vi "stage1.vi"() -> (0 "pass":bool=TRUE, 1 "Boolean 5":bool, 2 "Boolean 8":bool, 3 "Boolean 7":bool)   [LabVIEW 2014]
uses:
  <vilib>/Utility/miscctls.llb/LVPositionTypeDef.ctl
panel:
  out "star 3":bool
  out "star 2":bool
  out "star 1":bool
  out "result":bool
  in  "hh":dbl format="%0#2_6g"
  in  ":":dbl format="%0#2_6g"
  in  "ss":dbl format="%0#2_6g"
  in  "Position 2":T1={"Left"=876, "Top"=156}
  in  "Boolean 6":bool
  out "Boolean 3":bool
  out "Boolean":bool
  out "Boolean 2":bool
  in  "OK Button 43":bool
  in  "Position":T1
  in  "character":bool
  out "Map Array 2":bool[][](array[boolean])
  in  "Map Array":dbl[][](array[numeric])=array130x130[16900 elements]
  in  "OK Button 42":bool
  in  "OK Button 41":bool
  in  "OK Button 40":bool
  in  "OK Button 39":bool
  in  "OK Button 38":bool
  in  "OK Button 37":bool
  in  "OK Button 36":bool
  in  "OK Button 35":bool
  in  "OK Button 34":bool
  in  "OK Button 33":bool
  in  "OK Button 32":bool
  in  "OK Button 31":bool
  in  "OK Button 30":bool
  in  "OK Button 29":bool
  in  "OK Button 28":bool
  in  "OK Button 27":bool
  in  "OK Button 26":bool
  in  "OK Button 25":bool
  in  "OK Button 24":bool
  in  "OK Button 23":bool
  in  "OK Button 22":bool
  in  "OK Button 21":bool
  in  "stop 6":bool
  in  "OK Button 20":bool
  in  "OK Button 19":bool
  in  "OK Button 18":bool
  in  "OK Button 17":bool
  in  "OK Button 16":bool
  in  "OK Button 15":bool
  in  "OK Button 14":bool
  in  "OK Button 13":bool
  in  "OK Button 12":bool
  in  "OK Button 11":bool
  in  "stop 5":bool
  in  "stop 4":bool
  in  "OK Button 10":bool
  in  "OK Button 9":bool
  in  "OK Button 8":bool
  in  "OK Button 7":bool
  in  "OK Button 6":bool
  in  "OK Button 5":bool
  in  "stop 3":bool
  in  "stop 2":bool
  in  "stop":bool
  in  "OK Button 4":bool
  in  "OK Button 3":bool
  in  "OK Button 2":bool
  in  "OK Button":bool
  out "Boolean 4":bool
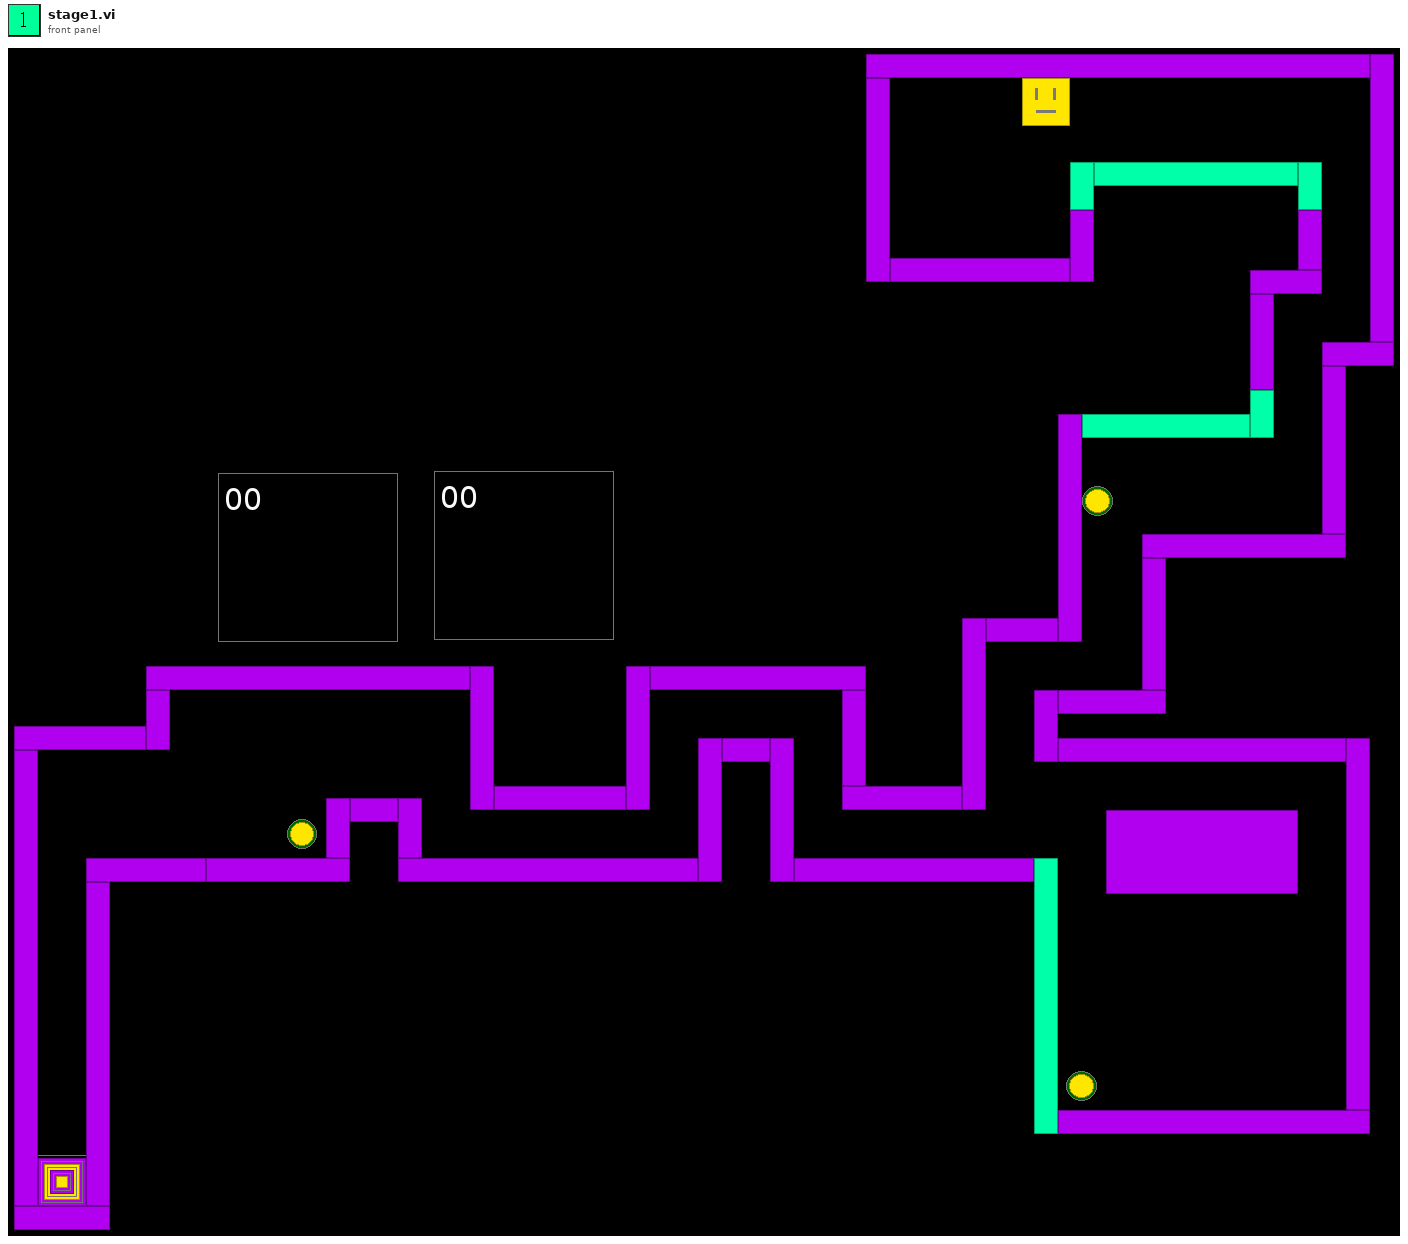
[diagram p1: front panel]
types:
  T1 = typedef "LVPositionTypeDef.ctl" = cluster{"Left":i32, "Top":i32}
  T2 = typedef "eventvkey.ctl" = enum16{"ASCII", "Enter", "Return", "Shift", "Ctrl", "Alt", "Cmd", "Opt", "Caps", "NumLock", "Clear", "Break", "Up", "Down", "Left", "Right", "Insert", "Delete", "Home", "End", "PageUp", "PageDown", "Escape", "Help", "Pause", "ScrollLock", "F1", "F2", "F3", "F4", "F5", "F6", "F7", "F8", "F9", "F10", "F11", "F12", "F13", "F14", "F15", "F16", "F17", "F18", "F19", "F20", "F21", "F22", "F23", "F24", "Play", "VolumeUp", "VolumeDown", "Mute", "Two Byte Char"}
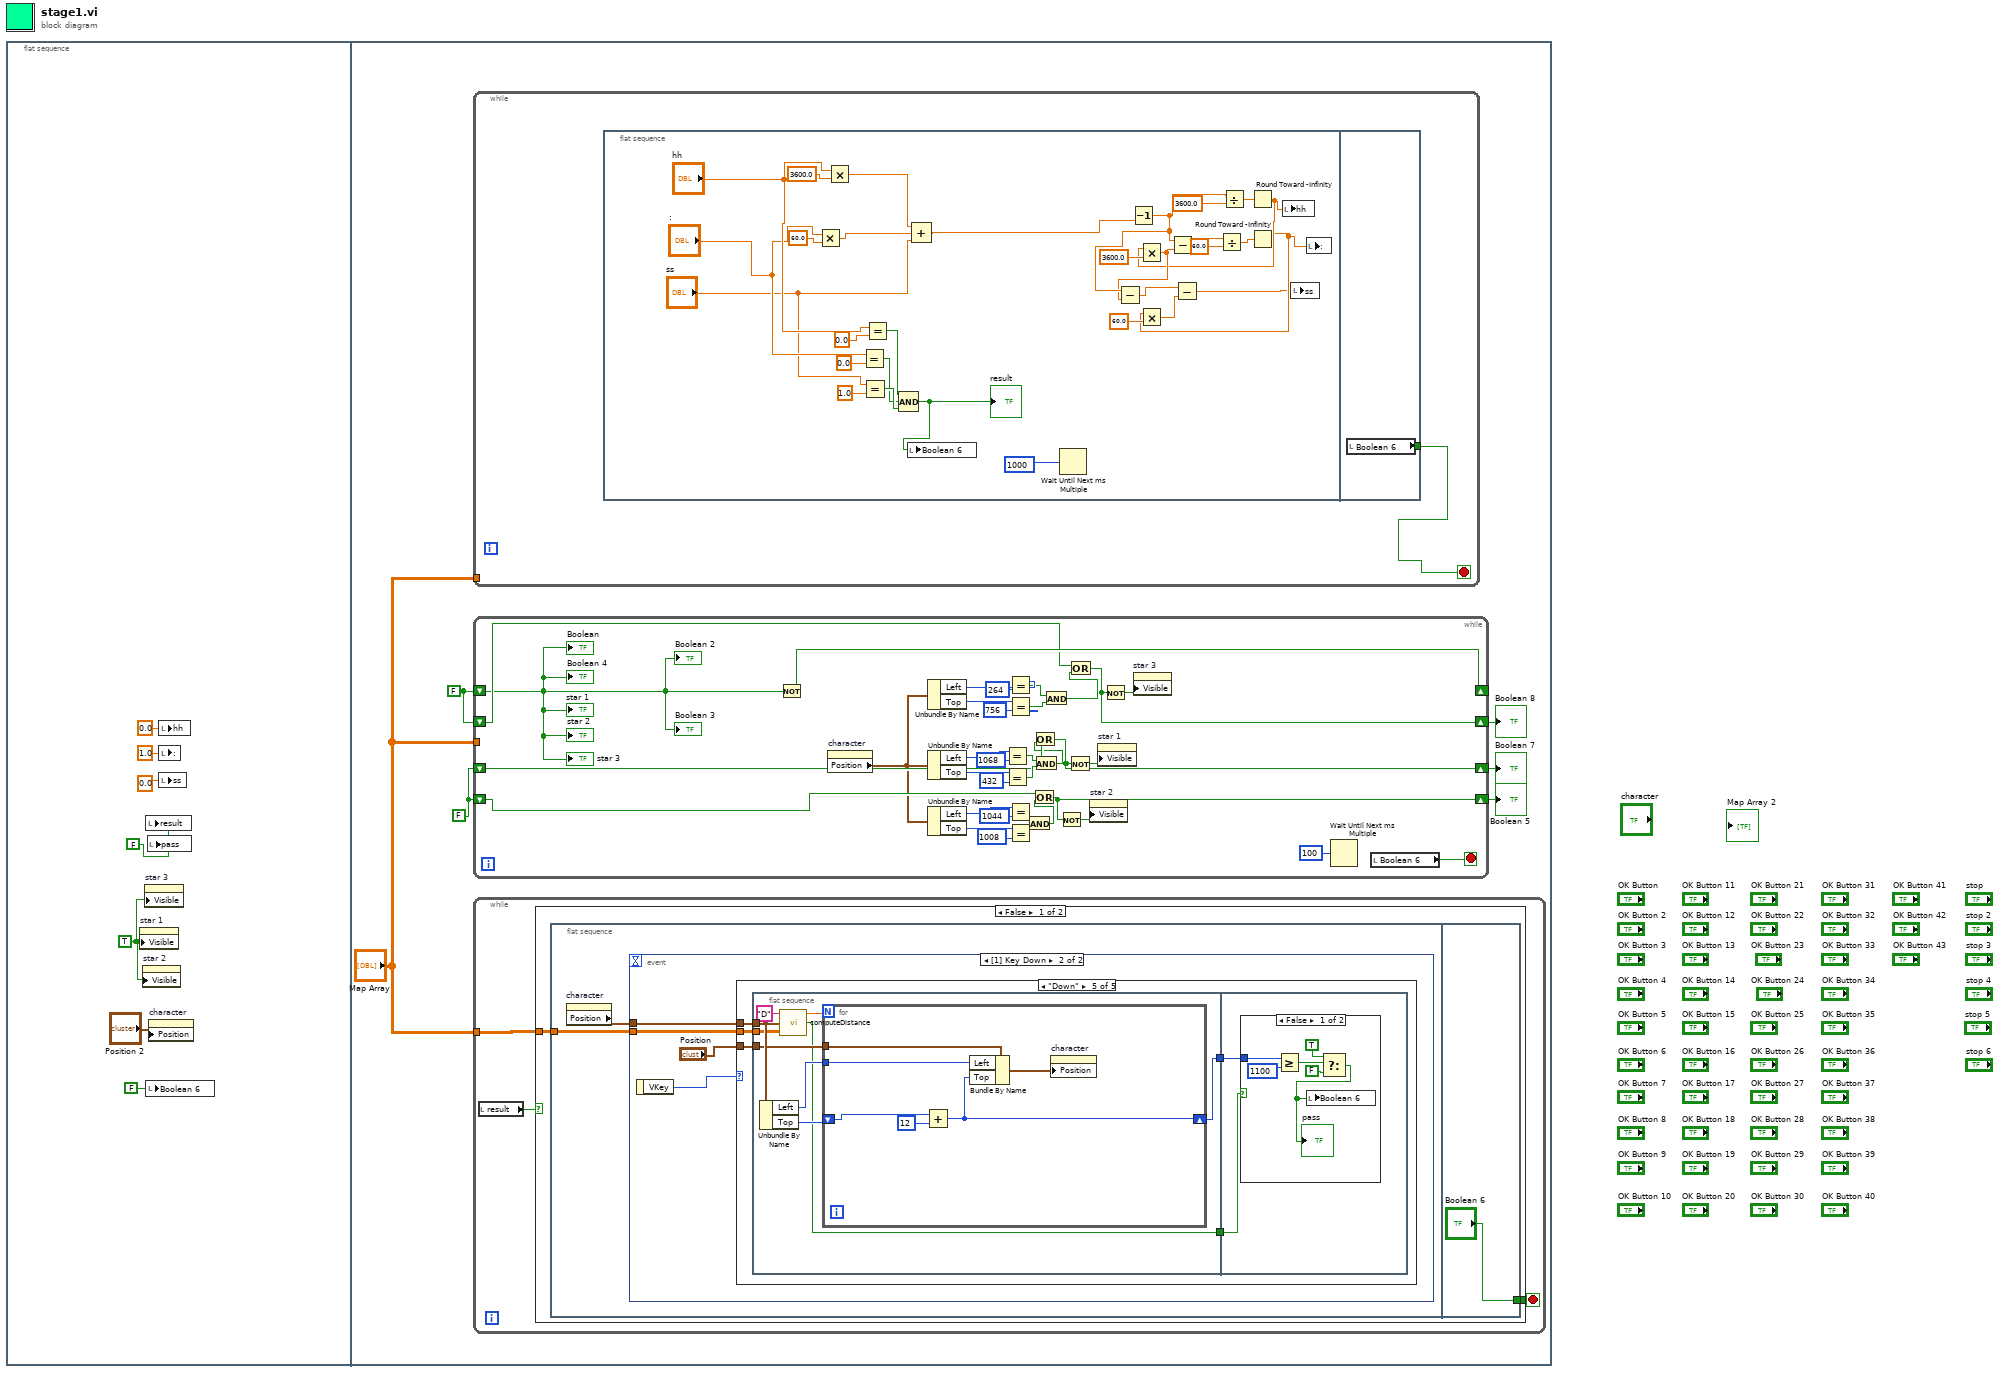
[diagram p0: block diagram]
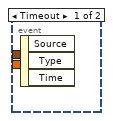
[diagram p2: hidden frame]
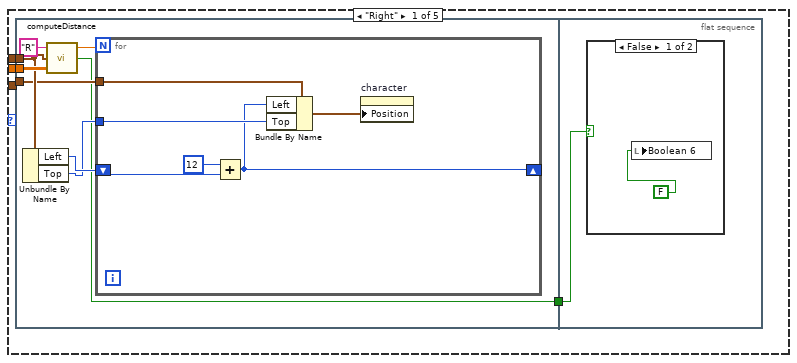
[diagram p3: hidden frame]
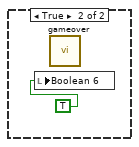
[diagram p4: hidden frame]
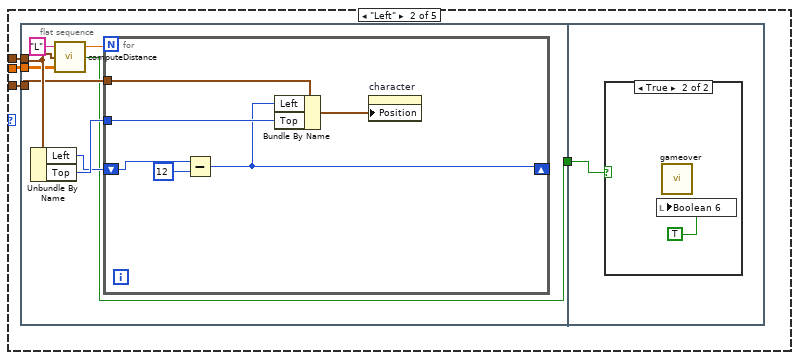
[diagram p5: hidden frame]
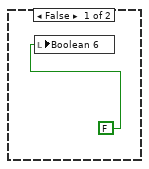
[diagram p6: hidden frame]
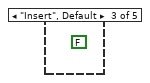
[diagram p7: hidden frame]
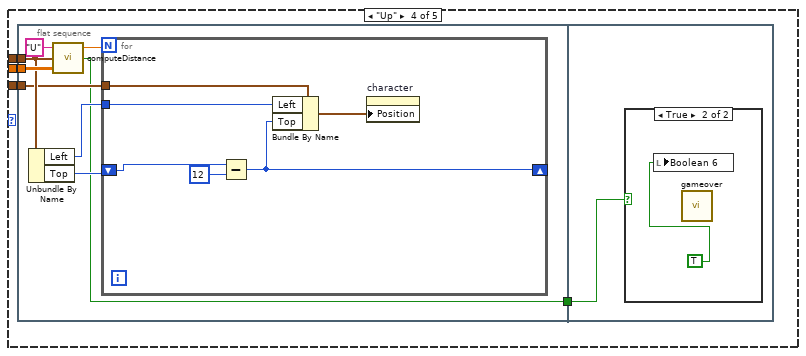
[diagram p8: hidden frame]
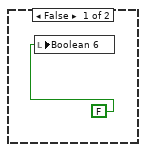
[diagram p9: hidden frame]
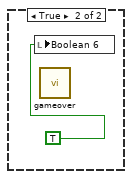
[diagram p10: hidden frame]
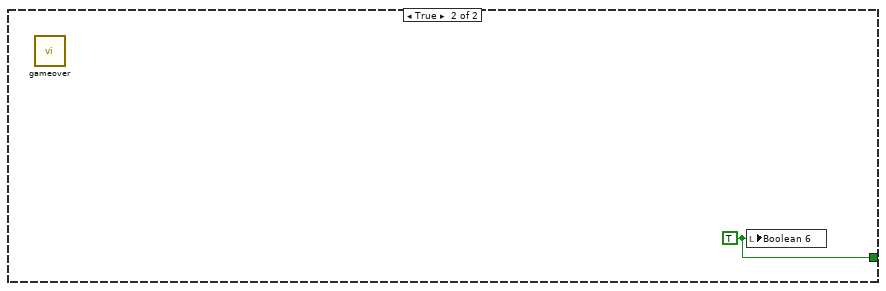
[diagram p11: hidden frame]
diagram:
  n1 = flat-sequence {
    frame #0 {
      w1 = TRUE ("Visible")
      w5 = FALSE ("star1")
      n2 = property on="star 1" class="Bool (strict)"("Visible"=w1) -> ()  [unwired: 2 in, 2 out]
      n3 = property on="star 2" class="Bool (strict)"("Visible"=w1) -> ()  [unwired: 2 in, 2 out]
      n4 = property on="star 3" class="Bool (strict)"("Visible"=w1) -> ()  [unwired: 2 in, 2 out]
      n5 = local write "result"(w5) -> ()
      n6 = local write "Boolean 6"(FALSE ("Boolean 6")) -> ()
      n7 = local write "pass"(w5) -> ()
      n8 = property on="character" class="Bool"("Position"="Position 2") -> ()  [unwired: 2 in, 2 out]
      n9 = local write "hh"(0.0 (":")) -> ()
      n10 = local write ":"(1.0 (":")) -> ()
      n11 = local write "ss"(0.0 ("ss")) -> ()
    }
    frame #1 {
      w12 = FALSE
      w11 = FALSE
      n12 = while {
        tunnel: "Map Array" -> [_]
        stop <- w14 stop-if-true
        n13 = flat-sequence {
          tunnel: [w45] -> w14
          frame #0 {
            n14 = Multiply(x=":", y=60.0) -> (x*y=w43:dbl)
            n15 = Multiply(x="hh", y=3600.0) -> (x*y=w44:dbl)
            n16 = Equal?(x=":", y=0.0) -> (x = y?=w35:bool)
            n17 = Equal?(x="ss", y=1.0) -> (x = y?=w36:bool)
            n18 = Equal?(x="hh", y=0.0) -> (x = y?=w34:bool)
            n19 = Compound Arithmetic op=AND(w34, w35, w36) -> (w15:bool)
            "result" <- w15
            n20 = local write "Boolean 6"(w15) -> ()
            n21 = Compound Arithmetic op=ADD(w44, w43, "ss") -> (w40:dbl)
            n22 = Wait Until Next ms Multiple(millisecond multiple=u32 1000) -> ()  [unwired: 1 out]
            n23 = Decrement(x=w40) -> (x-1=w29:dbl)
            n24 = Divide(x=w29, y=3600.0) -> (x/y=w19:dbl)
            n25 = Round Toward -Infinity(1:w19) -> (0:w18:dbl)
            n26 = Multiply(x=w18, y=3600.0) -> (x*y=w25:dbl)
            n27 = Subtract(x=w29, y=w25) -> (x-y=w26:dbl)
            n28 = Subtract(x=w29, y=w25) -> (x-y=w22:dbl)
            n29 = Divide(x=w22, y=60.0) -> (x/y=w24:dbl)
            n30 = Round Toward -Infinity(1:w24) -> (0:w17:dbl)
            n31 = Multiply(x=w17, y=60.0) -> (x*y=w28:dbl)
            n32 = Subtract(x=w26, y=w28) -> (x-y=w16:dbl)
            n33 = local write "hh"(w18) -> ()
            n34 = local write "ss"(w16) -> ()
            n35 = local write ":"(w17) -> ()
          }
          frame #1 {
            n36 = local read "Boolean 6"() -> (w45:bool)
          }
        }
      }
      n37 = while {
        shift-right: [w184] -> _
        shift-left: w11 -> [w151]
        tunnel: "Map Array" -> [_]
        shift-right: [w173] -> w9
        shift-left: w12 -> [w175]
        shift-right: [w164] -> w10
        shift-left: w12 -> [w163]
        shift-right: [w153] -> w8
        shift-left: w11 -> [w152]
        stop <- w183 stop-if-true
        n38 = Not(x=w151) -> (.not. x?=w184:bool)
        n39 = property on="character" class="Bool"() -> ("Position"=w154:T1)  [unwired: 2 in, 2 out]
        n40 = Unbundle By Name(w154) -> ("Left"=w162:i32, "Top"=w160:i32)
        n41 = Unbundle By Name(w154) -> ("Left"=w182:i32, "Top"=w180:i32)
        n42 = Unbundle By Name(w154) -> ("Left"=w165:i32, "Top"=w167:i32)
        n43 = Equal?(x=w182, y=1068) -> (x = y?=w178:bool)
        n44 = Equal?(x=w180, y=432) -> (x = y?=w177:bool)
        n45 = Equal?(x=w162, y=264) -> (x = y?=w158:bool)
        n46 = Equal?(x=w160, y=756) -> (x = y?=w157:bool)
        n47 = Equal?(x=w165, y=1044) -> (x = y?=w169:bool)
        n48 = Equal?(x=w167, y=1008) -> (x = y?=w170:bool)
        n49 = And(x=w169, y=w170) -> (x .and. y?=w172:bool)
        n50 = Or(x=w163, y=w172) -> (x .or. y?=w164:bool)
        n51 = And(x=w178, y=w177) -> (x .and. y?=w174:bool)
        n52 = Or(x=w175, y=w174) -> (x .or. y?=w173:bool)
        n53 = And(x=w158, y=w157) -> (x .and. y?=w155:bool)
        n54 = Not(x=w164) -> (.not. x?=w171:bool)
        n55 = Not(x=w173) -> (.not. x?=w176:bool)
        n56 = Or(x=w152, y=w155) -> (x .or. y?=w153:bool)
        n57 = property on="star 2" class="Bool (strict)"("Visible"=w171) -> ()  [unwired: 2 in, 2 out]
        n58 = property on="star 1" class="Bool (strict)"("Visible"=w176) -> ()  [unwired: 2 in, 2 out]
        n59 = Not(x=w153) -> (.not. x?=w156:bool)
        n60 = property on="star 3" class="Bool (strict)"("Visible"=w156) -> ()  [unwired: 2 in, 2 out]
        n61 = Wait Until Next ms Multiple(millisecond multiple=u32 100) -> ()  [unwired: 1 out]
        n62 = local read "Boolean 6"() -> (w183:bool)
        "Boolean" <- w151
        "Boolean 2" <- w151
        "Boolean 3" <- w151
        "Boolean 4" <- w151
        "star 1" <- w151
        "star 2" <- w151
        "star 3" <- w151
      }
      "Boolean 5" <- w10
      "Boolean 7" <- w9
      "Boolean 8" <- w8
      n63 = while {
        tunnel: "Map Array" -> [w48]
        stop <- w47 stop-if-true
        n64 = local read "result"() -> (w46:bool)
        n65 = case shown="False" w46 {
          tunnel: w48 -> [w50 _]
          tunnel: [w49 w150] -> w47
          frame False {
            n66 = flat-sequence {
              tunnel: w50 -> [w52]
              tunnel: ["Boolean 6"] -> w49
              frame #0 {
                n67 = property on="character" class="Bool"() -> ("Position"=w51:T1)  [unwired: 2 in, 2 out]
                n68 = event shown="[1] Key Down" {
                  selector: _ -> [_ _]
                  dyn-events: _ -> [_ _]
                  timeout: _ -> [_ _]
                  tunnel: w52 -> [_ w55]
                  tunnel: w51 -> [_ w54]
                  event Timeout {
                    n69 = event-data() -> ()  [unwired: 1 in, 3 out]
                  }
                  event Key Down {
                    n70 = event-data() -> ("VKey"=w56:T2)  [unwired: 1 in]
                    n71 = case shown="\"Down\"" w56 {
                      tunnel: w55 -> [w60 w80 _ w102 w123]
                      tunnel: w54 -> [w59 w81 _ w101 w124]
                      tunnel: "Position" -> [w58 w79 _ w100 w122]
                      frame "Right" {
                        n72 = flat-sequence {
                          tunnel: w60 -> [w66]
                          tunnel: w59 -> [w65]
                          tunnel: w58 -> [w64]
                          tunnel: [w61] -> w57
                          tunnel: w57 -> [w75]
                          frame #0 {
                            n73 = Unbundle By Name(w65) -> ("Left"=w63:i32, "Top"=w62:i32)
                            n74 = call "computeDistance.vi"("Array"=w66, "Position"=w65, "String"="R") -> ("2"=w61:bool, "distance"=w68:dbl)  [unwired: 1 out]
                            n75 = for {
                              N: w68 -> [_]
                              shift-right: [w71] -> _
                              shift-left: w63 -> [w74]
                              tunnel: w64 -> [w73]
                              tunnel: w62 -> [w72]
                              n76 = Add(x=12, y=w74) -> (x+y=w71:i32)
                              n77 = Bundle By Name(cluster=w73, "Left"=w71, "Top"=w72) -> (w69:T1)
                              n78 = property on="character" class="Bool"("Position"=w69) -> ()  [unwired: 2 in, 2 out]
                            }
                          }
                          frame #1 {
                            n79 = case shown="False" w75 {
                              frame False {
                                n80 = local write "Boolean 6"(FALSE) -> ()
                              }
                              frame True {
                                n81 = local write "Boolean 6"(TRUE) -> ()
                                n82 = call "gameover.vi"() -> ()  [unwired: 1 in]
                              }
                            }
                          }
                        }
                      }
                      frame "Left" {
                        n83 = flat-sequence {
                          tunnel: w81 -> [w85]
                          tunnel: w80 -> [w84]
                          tunnel: w79 -> [w83]
                          tunnel: [w82] -> w78
                          tunnel: w78 -> [w96]
                          frame #0 {
                            n84 = Unbundle By Name(w85) -> ("Left"=w88:i32, "Top"=w89:i32)
                            n85 = call "computeDistance.vi"("Array"=w84, "Position"=w85, "String"="L") -> ("2"=w82:bool, "distance"=w86:dbl)  [unwired: 1 out]
                            n86 = for {
                              N: w86 -> [_]
                              shift-right: [w93] -> _
                              shift-left: w88 -> [w92]
                              tunnel: w83 -> [w95]
                              tunnel: w89 -> [w94]
                              n87 = Subtract(x=w92, y=12) -> (x-y=w93:i32)
                              n88 = Bundle By Name(cluster=w95, "Left"=w93, "Top"=w94) -> (w90:T1)
                              n89 = property on="character" class="Bool"("Position"=w90) -> ()  [unwired: 2 in, 2 out]
                            }
                          }
                          frame #1 {
                            n90 = case shown="True" w96 {
                              frame False {
                                n91 = local write "Boolean 6"(FALSE) -> ()
                              }
                              frame True {
                                n92 = local write "Boolean 6"(TRUE) -> ()
                                n93 = call "gameover.vi"() -> ()  [unwired: 1 in]
                              }
                            }
                          }
                        }
                      }
                      frame "Insert", Default {
                        (unwired) FALSE
                      }
                      frame "Up" {
                        n94 = flat-sequence {
                          tunnel: w102 -> [w110]
                          tunnel: w101 -> [w107]
                          tunnel: w100 -> [w104]
                          tunnel: [w103] -> w99
                          tunnel: w99 -> [w117]
                          frame #0 {
                            n95 = Unbundle By Name(w107) -> ("Left"=w105:i32, "Top"=w106:i32)
                            n96 = call "computeDistance.vi"("Array"=w110, "Position"=w107, "String"="U") -> ("2"=w103:bool, "distance"=w108:dbl)  [unwired: 1 out]
                            n97 = for {
                              N: w108 -> [_]
                              shift-right: [w116] -> _
                              shift-left: w106 -> [w113]
                              tunnel: w105 -> [w115]
                              tunnel: w104 -> [w114]
                              n98 = Subtract(x=w113, y=12) -> (x-y=w116:i32)
                              n99 = Bundle By Name(cluster=w114, "Left"=w115, "Top"=w116) -> (w111:T1)
                              n100 = property on="character" class="Bool"("Position"=w111) -> ()  [unwired: 2 in, 2 out]
                            }
                          }
                          frame #1 {
                            n101 = case shown="True" w117 {
                              frame False {
                                n102 = local write "Boolean 6"(FALSE) -> ()
                              }
                              frame True {
                                n103 = local write "Boolean 6"(TRUE) -> ()
                                n104 = call "gameover.vi"() -> ()  [unwired: 1 in]
                              }
                            }
                          }
                        }
                      }
                      frame "Down" {
                        n105 = flat-sequence {
                          tunnel: w124 -> [w129]
                          tunnel: w123 -> [w128]
                          tunnel: w122 -> [w127]
                          tunnel: [w126] -> w121
                          tunnel: [w125] -> w120
                          tunnel: w121 -> [w141]
                          tunnel: w120 -> [w140]
                          frame #0 {
                            n106 = Unbundle By Name(w129) -> ("Left"=w133:i32, "Top"=w132:i32)
                            n107 = call "computeDistance.vi"("Array"=w128, "Position"=w129, "String"="D") -> ("2"=w126:bool, "distance"=w131:dbl)  [unwired: 1 out]
                            n108 = for {
                              N: w131 -> [_]
                              shift-right: [w139] -> w125
                              shift-left: w132 -> [w136]
                              tunnel: w133 -> [w138]
                              tunnel: w127 -> [w137]
                              n109 = Add(x=w136, y=12) -> (x+y=w139:i32)
                              n110 = Bundle By Name(cluster=w137, "Left"=w138, "Top"=w139) -> (w134:T1)
                              n111 = property on="character" class="Bool"("Position"=w134) -> ()  [unwired: 2 in, 2 out]
                            }
                          }
                          frame #1 {
                            n112 = case shown="False" w141 {
                              tunnel: w140 -> [w147 _]
                              frame False {
                                n113 = Greater Or Equal?(x=w147, y=1100) -> (x >= y?=w145:bool)
                                n114 = Select(t=TRUE, s=w145, f=FALSE) -> (s? t:f=w142:bool)
                                "pass" <- w142
                                n115 = local write "Boolean 6"(w142) -> ()
                              }
                              frame True {
                                n116 = local write "Boolean 6"(TRUE) -> ()
                                n117 = call "gameover.vi"() -> ()  [unwired: 1 in]
                              }
                            }
                          }
                        }
                      }
                    }
                  }
                }
              }
              frame #1 {
              }
            }
          }
          frame True {
            w150 = TRUE ("Boolean 6")
            n118 = call "gameover.vi"() -> ()  [unwired: 1 in]
            n119 = local write "Boolean 6"(w150) -> ()
          }
        }
      }
    }
  }
